vi "Receive Value.vi"(10 "Numeric":dbl, 11 "Caller in":refnum<class "Caller A.lvclass">) -> (3 "Caller out":refnum<class "Caller A.lvclass">)   [LabVIEW 2023, in "Caller A.lvlib" / "Caller A.lvclass"]
uses:
  Caller A.lvclass
  Caller A.lvclass/Caller A.ctl
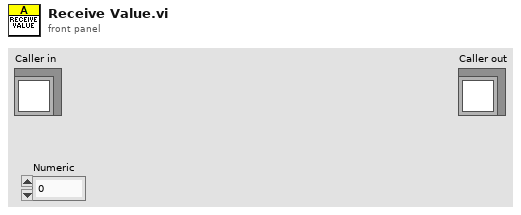
[diagram p1: front panel]
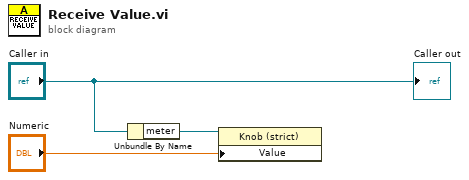
[diagram p0: block diagram]
diagram:
  n1 = Unbundle By Name("Caller in") -> ("meter"=w2:refnum<vi>)
  n2 = property class="Knob (strict)"(reference=w2, "Value"="Numeric") -> ()  [unwired: 1 in, 2 out]
  "Caller out" <- "Caller in"
